vi "SAC-Build Filename.vi"(0 "State":T1) -> (4 "path":path, 8 "filestem":string)   [LabVIEW 2020]
uses:
  Typedefs/SAC-State.ctl
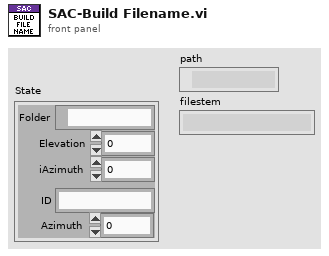
[diagram p1: front panel]
types:
  T1 = typedef "SAC-State.ctl" = cluster{"Folder":path, "Elevation":dbl, "iAzimuth":i32, "ID":string, "Azimuth":dbl}
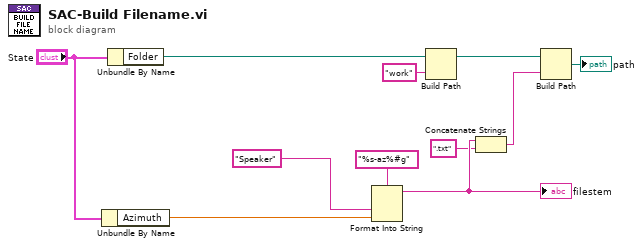
[diagram p0: block diagram]
diagram:
  n1 = Unbundle By Name("State") -> ("Azimuth"=w4:dbl)
  n2 = Unbundle By Name("State") -> ("Folder"=w8:path)
  n3 = Format Into String(format string="%s-az%#g", "Speaker", w4) -> (resulting string=w3:string)  [unwired: 2 in, 1 out]
  "filestem" <- w3
  n4 = Build Path(base path=w8, name or relative path="work") -> (appended path=w6:path)
  n5 = Concatenate Strings(w3, ".txt" ("format string")) -> (w1:string)
  n6 = Build Path(base path=w6, name or relative path=w1) -> (appended path=→"path":path)
